vi "RT Sound.vi"(8 "error in":errorcluster, 9 "Sound Options":T1, 10 "Volume":fxp<+/-,32,16>=0.5, 11 "FPGA VI Reference In":refnum<k20>) -> (0 "error out":errorcluster, 3 "FPGA VI Reference Out":refnum<k20>)   [LabVIEW 2016]
doc: "This VI plays an alarm sound through the speaker by utilizing the analog output on the board.\n\nEach alarm sound is stored in a pre-built array containing waveform data. This data is streamed to the FPGA and then out through the analog output. Before the waveform is streamed, the gain of the output must be set. The waveform data is multiplied by this value, allowing for volume control. The RT-FPGA DMA FIFO must also be configured to be large enough to allow seamless data stream."
uses:
  controls/SoundOptions.ctl
  <vilib>/Utility/error.llb/Error Cluster From Error Code.vi
  <vilib>/rvi/errors/niLvFpgaAdjustHostInterfaceError.vi
  <vilib>/rvi/interface/common/niFpgaWaitOnOcc.vi
  <vilib>/rvi/interface/nirviReadWriteControl/nirviReadWriteControl.xnode
  <vilib>/rvi/interface/nirviMethod/nirviMethod.xnode
  <vilib>/rvi/errors/niLvFpgaMergeErrorWithErrorCode.vi
  NiFpgaLv.dll
  <vilib>/rvi/interface/Simulation/niFpgaSimulationCallBeginRW.vi
  <vilib>/FPGAPlugInAG/Dynamic/niLvFpga_ConfigureFifo_Dynamic.vi
  <vilib>/FPGAPlugInAG/Dynamic/niLvFpga_WriteFifo_Dynamic.vi
panel:
  # "Recommended value \nfor gain is around .5"
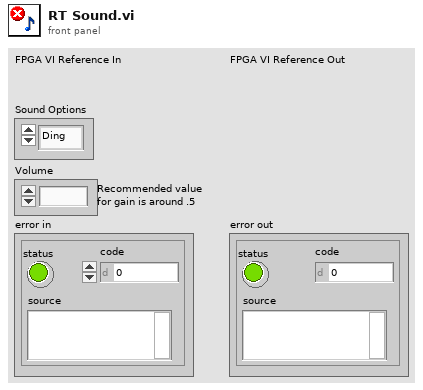
[diagram p1: front panel]
types:
  T1 = typedef "SoundOptions.ctl" = enum16{"Ding", "Boing", "Buzzer", "Horn"}
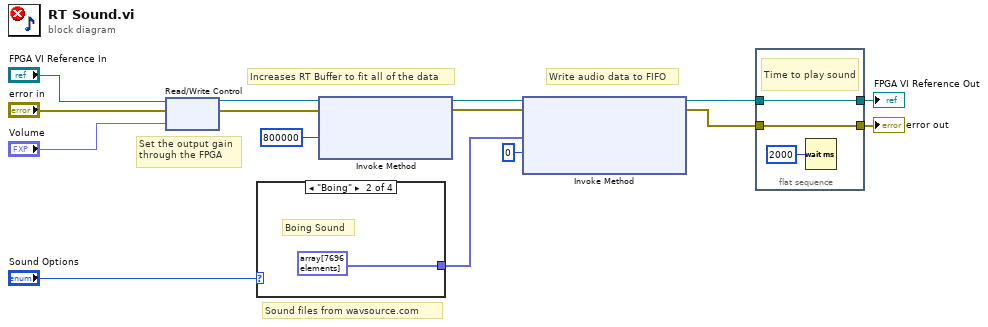
[diagram p0: block diagram]
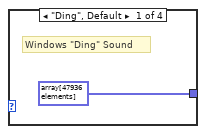
[diagram p2: hidden frame]
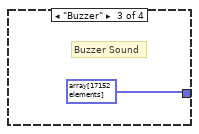
[diagram p3: hidden frame]
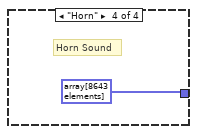
[diagram p4: hidden frame]
diagram:
  # "Set the output gain\nthrough the FPGA"
  # "Sound files from wavsource.com"
  # "Increases RT Buffer to fit all of the data"
  # "Write audio data to FIFO"
  n1 = xnode "Read/Write Control"("FPGA VI Reference In"="FPGA VI Reference In", "error in"="error in", "Gain"="Volume") -> ("FPGA VI Reference Out"=w11:refnum<k20>, "error out"=w10:errorcluster)
  n2 = case shown="\"Boing\"" "Sound Options" {
    tunnel: [fxp<+/-,32,16>[] array[47936 elements] ("Array") fxp<+/-,32,16>[] array[7696 elements] ("Array") fxp<+/-,32,16>[] array[17152 elements] ("Array") fxp<+/-,32,16>[] array[8643 elements] ("Array")] -> w6
    frame "Ding", Default {
      # "Windows \"Ding\" Sound"
    }
    frame "Boing" {
      # "Boing Sound"
    }
    frame "Buzzer" {
      # "Buzzer Sound"
    }
    frame "Horn" {
      # "Horn Sound"
    }
  }
  n3 = xnode "Invoke Method"("FPGA VI Reference In"=w11, "error in"=w10, "Requested Depth"=u32 800000) -> ("FPGA VI Reference Out"=w9:refnum<k20>, "error out"=w8:errorcluster)  [unwired: 1 out]
  n4 = xnode "Invoke Method"("FPGA VI Reference In"=w9, "error in"=w8, "Data"=w6, "Timeout (ms)"=0 ("Timeout")) -> ("FPGA VI Reference Out"=w5:refnum<k20>, "error out"=w4:errorcluster)  [unwired: 1 out]
  n5 = flat-sequence {
    tunnel: w4 -> [w22]
    tunnel: [w22] -> w12
    tunnel: w5 -> [w21]
    tunnel: [w21] -> w1
    frame #0 {
      # "Time to play sound"
      n6 = Wait (ms)(milliseconds to wait=u32 2000) -> ()  [unwired: 1 out]
    }
  }
  "error out" <- w12
  "FPGA VI Reference Out" <- w1
